vi "PasswordPrompt.vi"() -> (1 "OK?":bool)   [LabVIEW 2026]
uses:
  C:/Users/bjames/Documents/GitHub/LVAutomation/Support Files/VarexLib.dll
  Support Files/VarexLib.dll
panel:
  out "String":string
  in  "Cancel":bool
  in  "OK":bool
  in  "Password":string
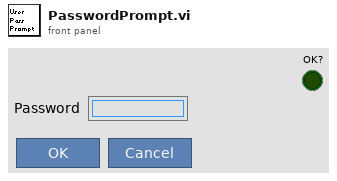
[diagram p1: front panel]
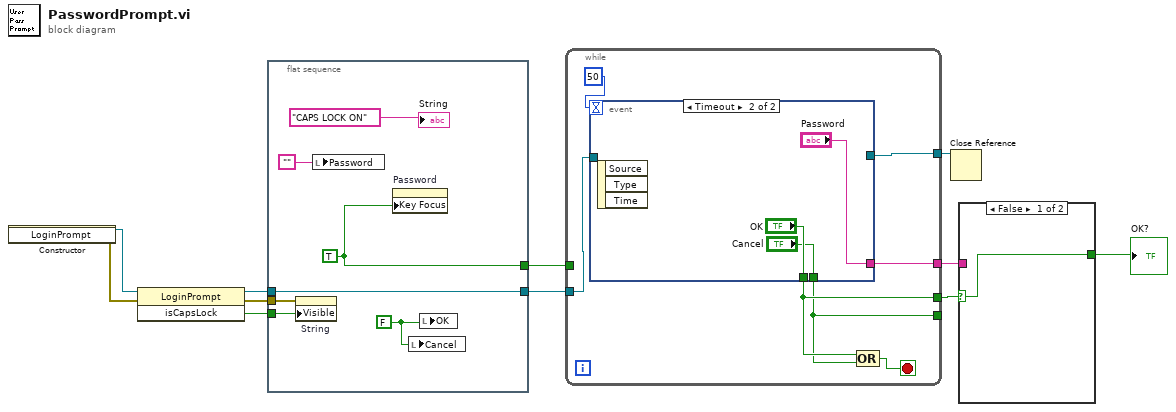
[diagram p0: block diagram]
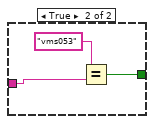
[diagram p2: hidden frame]
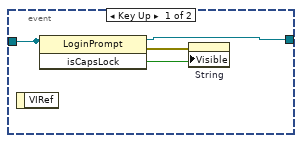
[diagram p3: hidden frame]
diagram:
  n1 = constructor class="LoginPrompt"() -> (reference out=w2:refnum<k24>, error out=w1:errorcluster)  [unwired: 3 in, 1 out]
  n2 = invoke class="LoginPrompt" method="isCapsLock"(reference=w2, error in=w1) -> (reference out=w6:refnum<k24>, error out=w5:errorcluster, "isCapsLock"=w7:bool)  [unwired: 1 in]
  n3 = flat-sequence {
    tunnel: [w16] -> w11
    tunnel: w7 -> [w15]
    tunnel: w6 -> [w13]
    tunnel: w5 -> [w14]
    tunnel: [w13] -> w4
    frame #0 {
      w17 = FALSE
      w16 = TRUE
      n4 = property on="String" class="Str"(error in=w14, "Visible"=w15) -> ()  [unwired: 1 in, 2 out]
      n5 = local write "Password"("") -> ()
      n6 = property on="Password" class="Str"("Key Focus"=w16) -> ()  [unwired: 2 in, 2 out]
      n7 = local write "Cancel"(w17) -> ()
      n8 = local write "OK"(w17) -> ()
      "String" <- "CAPS LOCK ON"
    }
  }
  n9 = while {
    tunnel: w11 -> [_]
    tunnel: [w21] -> w10
    tunnel: [w20] -> _
    tunnel: [w22] -> w9
    tunnel: w4 -> [w24]
    tunnel: [w23] -> w3
    stop <- w25 stop-if-true
    n10 = event shown="[1] Timeout" {
      selector: _ -> [_ _]
      dyn-events: _ -> [_ _]
      timeout: u32 50 ("milliseconds to wait") -> [_ _]
      tunnel: [w29 _] -> _
      tunnel: w24 -> [w29 _]
      tunnel: [w26 _] -> w23
      tunnel: [_ "Password"] -> w22
      tunnel: [_ "OK"] -> w21
      tunnel: [_ "Cancel"] -> w20
      event Key Up {
        n11 = event-data() -> ()  [unwired: 1 in, 1 out]
        n12 = invoke class="LoginPrompt" method="isCapsLock"(reference=w29) -> (reference out=w26:refnum<k24>, error out=w27:errorcluster, "isCapsLock"=w28:bool)  [unwired: 2 in]
        n13 = property on="String" class="Str"(error in=w27, "Visible"=w28) -> ()  [unwired: 1 in, 2 out]
      }
      event Timeout {
        n14 = event-data() -> ()  [unwired: 1 in, 3 out]
      }
    }
    n15 = Compound Arithmetic op=OR(w21, w20) -> (w25:bool)
  }
  n16 = Close Reference(reference=w3) -> ()  [unwired: 1 in, 1 out]
  n17 = case shown="False" w10 {
    selector: w10 -> [w33 _]
    tunnel: w9 -> [_ w35]
    tunnel: [w33 w34] -> w8
    frame False {
    }
    frame True {
      n18 = Equal?(x="vms053", y=w35) -> (x = y?=w34:bool)
    }
  }
  "OK?" <- w8
